vi "dfd_Expand Filter Quantizers.vi"(11 "FXPOPs":T1[](array[typedef]) {"source" items=["Coef a/k"=0, "Coef b/v"=7, "Input"=1, "Output"=2, "Multiplicand"=3, "Product"=4, "Sum"=5, "Delay"=6, "Gain"=8]}) -> (0 "Delay":T1={"source"=0, "is floating?"=FALSE, "o-mode"=enum."Wrap", "q-mode"=enum."Nearest", "signed?"=FALSE, "fwl"=0, "high limit"=0.0, "low limit"=0.0, "full range"=0.0} {"source" items=["Coef a/k"=0, "Coef b/v"=7, "Input"=1, "Output"=2, "Multiplicand"=3, "Product"=4, "Sum"=5, "Delay"=6, "Gain"=8]}, 1 "Sum":T1={"source"=0, "is floating?"=FALSE, "o-mode"=enum."Wrap", "q-mode"=enum."Nearest", "signed?"=FALSE, "fwl"=0, "high limit"=0.0, "low limit"=0.0, "full range"=0.0} {"source" items=["Coef a/k"=0, "Coef b/v"=7, "Input"=1, "Output"=2, "Multiplicand"=3, "Product"=4, "Sum"=5, "Delay"=6, "Gain"=8]}, 2 "Product":T1={"source"=0, "is floating?"=FALSE, "o-mode"=enum."Wrap", "q-mode"=enum."Nearest", "signed?"=FALSE, "fwl"=0, "high limit"=0.0, "low limit"=0.0, "full range"=0.0} {"source" items=["Coef a/k"=0, "Coef b/v"=7, "Input"=1, "Output"=2, "Multiplicand"=3, "Product"=4, "Sum"=5, "Delay"=6, "Gain"=8]}, 3 "Multiplicand":T1={"source"=0, "is floating?"=FALSE, "o-mode"=enum."Wrap", "q-mode"=enum."Nearest", "signed?"=FALSE, "fwl"=0, "high limit"=0.0, "low limit"=0.0, "full range"=0.0} {"source" items=["Coef a/k"=0, "Coef b/v"=7, "Input"=1, "Output"=2, "Multiplicand"=3, "Product"=4, "Sum"=5, "Delay"=6, "Gain"=8]}, 4 "Coefficient b/v":T1={"source"=0, "is floating?"=FALSE, "o-mode"=enum."Wrap", "q-mode"=enum."Truncation", "signed?"=FALSE, "fwl"=0, "high limit"=0.0, "low limit"=0.0, "full range"=0.0} {"source" items=["Coef a/k"=0, "Coef b/v"=7, "Input"=1, "Output"=2, "Multiplicand"=3, "Product"=4, "Sum"=5, "Delay"=6, "Gain"=8]}, 5 "Output":T1={"source"=0, "is floating?"=FALSE, "o-mode"=enum."Wrap", "q-mode"=enum."Nearest", "signed?"=FALSE, "fwl"=0, "high limit"=0.0, "low limit"=0.0, "full range"=0.0} {"source" items=["Coef a/k"=0, "Coef b/v"=7, "Input"=1, "Output"=2, "Multiplicand"=3, "Product"=4, "Sum"=5, "Delay"=6, "Gain"=8]}, 6 "Coefficient a/k":T1={"source"=0, "is floating?"=FALSE, "o-mode"=enum."Wrap", "q-mode"=enum."Nearest", "signed?"=FALSE, "fwl"=0, "high limit"=0.0, "low limit"=0.0, "full range"=0.0} {"source" items=["Coef a/k"=0, "Coef b/v"=7, "Input"=1, "Output"=2, "Multiplicand"=3, "Product"=4, "Sum"=5, "Delay"=6, "Gain"=8]}, 7 "Input":T1={"source"=0, "is floating?"=FALSE, "o-mode"=enum."Wrap", "q-mode"=enum."Nearest", "signed?"=FALSE, "fwl"=0, "high limit"=0.0, "low limit"=0.0, "full range"=0.0} {"source" items=["Coef a/k"=0, "Coef b/v"=7, "Input"=1, "Output"=2, "Multiplicand"=3, "Product"=4, "Sum"=5, "Delay"=6, "Gain"=8]}, 8 "Gain":T1={"source"=0, "is floating?"=FALSE, "o-mode"=enum."Wrap", "q-mode"=enum."Truncation", "signed?"=FALSE, "fwl"=0, "high limit"=0.0, "low limit"=0.0, "full range"=0.0} {"source" items=["Coef a/k"=0, "Coef b/v"=7, "Input"=1, "Output"=2, "Multiplicand"=3, "Product"=4, "Sum"=5, "Delay"=6, "Gain"=8]})   [LabVIEW 2017, in "NI_DigFilter_FXP.lvlib"]
uses:
  <vilib>/addons/Digital Filter Design/NI_DigFilter_FXP.lvlib
  <vilib>/addons/Digital Filter Design/_Objects.llb/dfd_FXP Operation.ctl
  <vilib>/addons/Digital Filter Design/_Objects.llb/dfd_Internal Quantization Srcs.ctl
  <vilib>/addons/Digital Filter Design/NI_DigFilterLicensed.lvlib
types:
  T1 = typedef "dfd_FXP Operation.ctl" = cluster{"source":T2, "is floating?":bool, "o-mode":enum16{"Saturation", "Wrap"}, "q-mode":enum16{"Nearest", "Truncation"}, "signed?":bool, "fwl":i16, "high limit":ext, "low limit":ext, "full range":ext}
  T2 = typedef "NI_DigFilterLicensed.lvlib/dfd_Internal Quantization Srcs.ctl" = u16
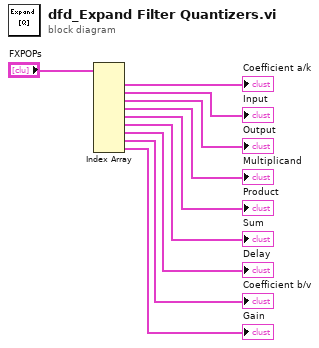
[diagram p0: block diagram]
diagram:
  n1 = Index Array(array="FXPOPs") -> (element #1=→"Coefficient a/k":T1, element #2=→"Input":T1, element #3=→"Output":T1, element #4=→"Multiplicand":T1, element #5=→"Product":T1, element #6=→"Sum":T1, element #7=→"Delay":T1, element #8=→"Coefficient b/v":T1, element #9=→"Gain":T1)  [unwired: 9 in]
